vi "Close.vi"(8 "error in (no error)":errorcluster, 11 "Shadow in":refnum<class "Shadow.lvclass">) -> (0 "error out":errorcluster, 3 "Shadow out":refnum<class "Shadow.lvclass">)   [LabVIEW 2021, in "UIShadow.lvlib" / "Shadow.lvclass"]
uses:
  Shadow.lvclass
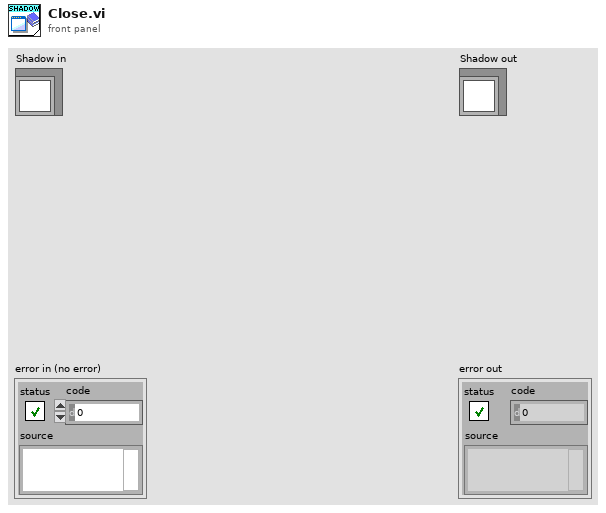
[diagram p1: front panel]
types:
  T1 = typedef "UIShadow.lvlib/Shadow.lvclass/Data.ctl" = cluster{"VI Refnum":refnum<vi>, "ShadowColor":u32, "Offset":i16, "Transparancy":i32, "UIShadowRef":refnum<vi>, "Activate?":bool}
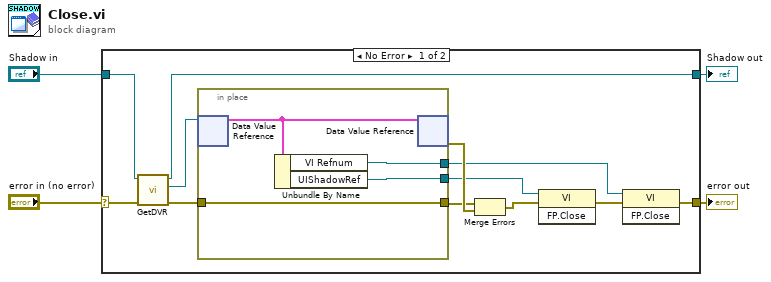
[diagram p0: block diagram]
diagram:
  n1 = case shown="No Error" "error in (no error)" {
    selector: "error in (no error)" -> [w16 w22]
    tunnel: [w6 w22] -> w3
    tunnel: [w15 w21] -> w1
    tunnel: "Shadow in" -> [w14 w21]
    frame No Error {
      n2 = call "GetDVR.vi"("error in (no error)"=w16, "Shadow in"=w14) -> ("error out"=w10:errorcluster, "DVR"=w11:refnum<data-value>, "Shadow out"=w15:refnum<class "Shadow.lvclass">)  [unwired: 7 in]
      n3 = in-place {
        in-place-border: w10 -> [w20]
        in-place-border: [w20] -> w12
        in-place-border: [w18] -> w5
        in-place-border: [w17] -> w8
        n4 = in-place-dvr #1(w11) -> (w19:T1)  [unwired: 1 out]
        n5 = Unbundle By Name(w19) -> ("VI Refnum"=w18:refnum<vi>, "UIShadowRef"=w17:refnum<vi>)
        n6 = in-place-dvr #1(w19) -> (w13:errorcluster)  [unwired: 1 out]
      }
      n7 = Merge Errors(w12, w13) -> (w9:errorcluster)
      n8 = invoke class="VI" method="FP.Close"(reference=w8, error in=w9) -> (error out=w7:errorcluster)  [unwired: 1 in, 2 out]
      n9 = invoke class="VI" method="FP.Close"(reference=w5, error in=w7) -> (error out=w6:errorcluster)  [unwired: 1 in, 2 out]
    }
    frame Error {
    }
  }
  "error out" <- w3
  "Shadow out" <- w1
